vi "ma_SML Decimation Filter.vi"   [LabVIEW 2020, in "NI_MAPro.lvlib"]
uses:
  NI_MAPro.lvlib
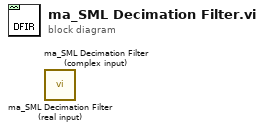
[diagram p0: block diagram]
diagram:
  n1 = call "ma_SML Decimation Filter (real input).vi"() -> ()  [unwired: 4 in, 2 out]
  n2 = call "ma_SML Decimation Filter (complex input).vi"() -> ()  [unwired: 4 in, 2 out]
